vi "getChannelList Modify.vi"(4 "error in (no error)":errorcluster, 5 "channel names":string, 6 "group name":string, 7 "tdms file":refnum<k34>) -> (0 "error out":errorcluster, 1 "channel names out":string[](array[string]), 2 "group names out":string[](array[string]), 3 "tdms file out":refnum<k34>)   [LabVIEW 2012]
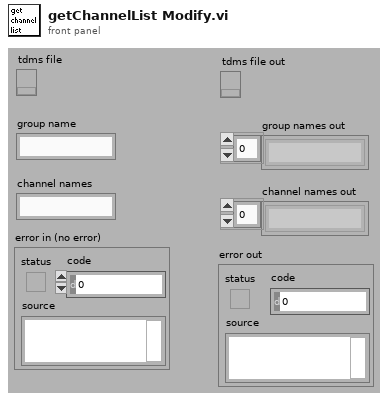
[diagram p1: front panel]
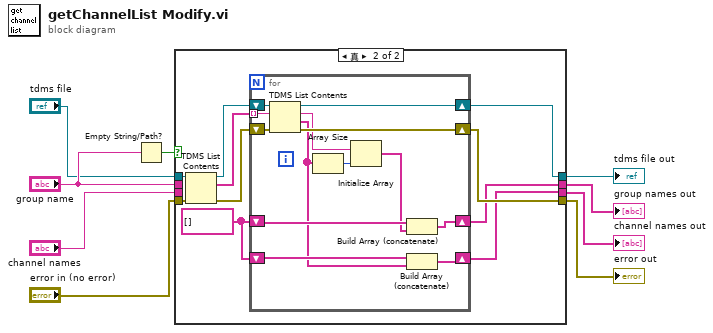
[diagram p0: block diagram]
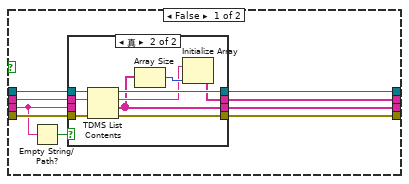
[diagram p2: hidden frame]
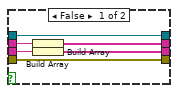
[diagram p3: hidden frame]
diagram:
  n1 = Empty String/Path?(string/path="group name") -> (empty?=w7:bool)
  n2 = case shown="真" w7 {
    tunnel: "tdms file" -> [w17 w43]
    tunnel: "error in (no error)" -> [w16 w42]
    tunnel: "channel names" -> [w15 _]
    tunnel: [w14 w37] -> w4
    tunnel: [w13 w39] -> w5
    tunnel: [w12 w34] -> w6
    tunnel: "group name" -> [w11 _]
    tunnel: [w10 w35] -> w9
    frame False {
      n3 = Empty String/Path?(string/path=w15) -> (empty?=w18:bool)
      n4 = case shown="真" w18 {
        tunnel: w17 -> [w23 w33]
        tunnel: w16 -> [w24 w32]
        tunnel: [w24 w31] -> w14
        tunnel: [w23 w30] -> w13
        tunnel: w11 -> [w20 w29]
        tunnel: [w21 w25] -> w12
        tunnel: w15 -> [w22 _]
        tunnel: [w19 w26] -> w10
        frame False {
          n5 = Build Array(w20) -> (w19:string[])
          n6 = Build Array(w22) -> (w21:string[])
        }
        frame True {
          n7 = TDMS List Contents(4:w32, 6:w29, 7:w33) -> (0:w31:errorcluster, 1:w25:string[], 2:w27:string, 3:w30:refnum<k34>)
          n8 = Array Size(array=w25) -> (size(s)=w28:i32)
          n9 = Initialize Array(w27, w28) -> (w26:string[])
        }
      }
    }
    frame True {
      w36 = string[] [] ("组名称")
      n10 = TDMS List Contents(4:w42, 7:w43) -> (0:w38:errorcluster, 2:w41:string[], 3:w40:refnum<k34>)  [unwired: 1 in, 1 out]
      n11 = for {
        tunnel: w41 -> [w56] mode=indexing
        shift-right: [w54] -> w39
        shift-left: w40 -> [w55]
        shift-right: [w52] -> w37
        shift-left: w38 -> [w53]
        shift-right: [w47] -> w35
        shift-left: w36 -> [w49]
        shift-right: [w44] -> w34
        shift-left: w36 -> [w46]
        n12 = TDMS List Contents(4:w53, 6:w56, 7:w55) -> (0:w52:errorcluster, 1:w45:string[], 2:w51:string, 3:w54:refnum<k34>)
        n13 = Array Size(array=w45) -> (size(s)=w50:i32)
        n14 = Initialize Array(w51, w50) -> (w48:string[])
        n15 = Build Array (concatenate)(w49, w48) -> (w47:string[])
        n16 = Build Array (concatenate)(w46, w45) -> (w44:string[])
      }
    }
  }
  "group names out" <- w9
  "channel names out" <- w6
  "tdms file out" <- w5
  "error out" <- w4
